vi "Stop Core.vi"(10 "final error code":i32, 11 "SoftwareSetup In":refnum<class "SoftwareSetup.lvclass">) -> (3 "SoftwareSetup Out":refnum<class "SoftwareSetup.lvclass">)   [LabVIEW 2019, in "SoftwareSetup.lvlib" / "SoftwareSetup.lvclass"]
uses:
  SoftwareSetup.lvclass
  SoftwareSetup.lvclass/SoftwareSetup.ctl
  SystemSetup/SystemSetup/SystemSetup.lvclass
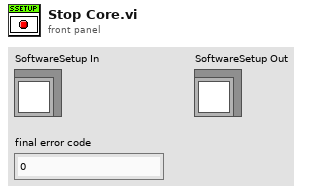
[diagram p1: front panel]
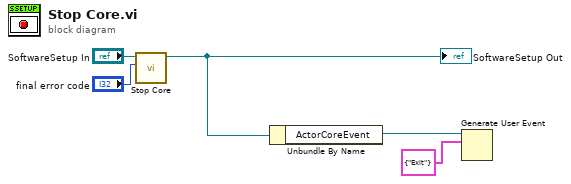
[diagram p0: block diagram]
diagram:
  n1 = call-parent "Stop Core.vi"("final error code"="final error code", "Event Source In"="SoftwareSetup In") -> ("Event Source Out"=w3:refnum<class "SoftwareSetup.lvclass">)  [unwired: 9 in]
  "SoftwareSetup Out" <- w3
  n2 = Unbundle By Name(w3) -> ("ActorCoreEvent"=w2:refnum<user-event>)
  n3 = Generate User Event(user event=w2, event data cluster=cluster{"ActorCoreMessage":string} {"ActorCoreMessage"="Exit"} ("event data")) -> ()  [unwired: 2 in, 2 out]
